vi "python_test2_quadarrays 1.vi"(0 "Time Array":dbl[](array[numeric]), 1 "Python Path on host machine":path=path "C:/Program Files (x86)/Python39-32/python.exe", 2 "Python Module Path on host machine":path=path "C:/Users/idewe/Projects/LabviewProjects/Sonomatic SQLite3 Testing/add_2_nums.py", 5 "Press Array":dbl[](array[numeric]), 7 "Temp Array":dbl[](array[numeric]), 9 "Dens Array":dbl[](array[numeric]), 11 "error in (no error)":errorcluster, 12 "Python_Function_Name":string="sum_function", 13 "Python Version":string="3.9.2") -> (4 "Python Numeric Output":dbl[](array[numeric]), 15 "error out":errorcluster)   [LabVIEW 2023]
panel:
  # "PYTHON METHOD CALL EXAMPLE"
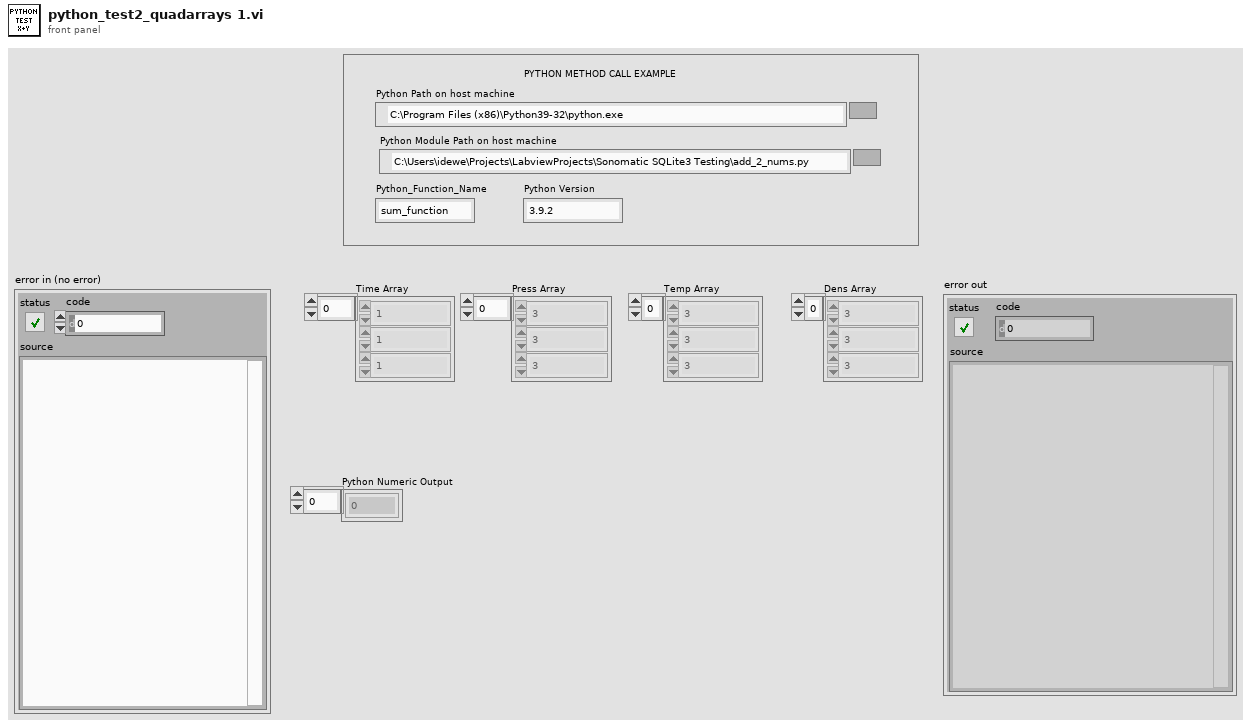
[diagram p1: front panel]
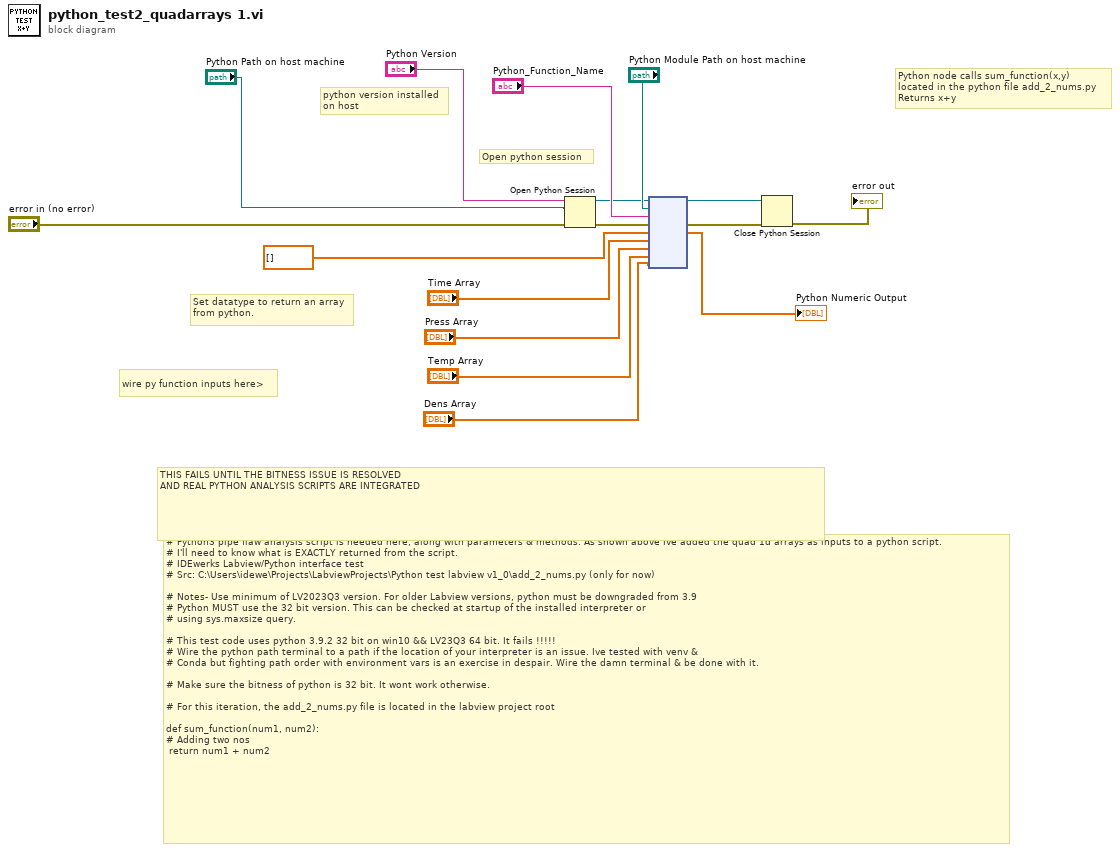
[diagram p0: block diagram]
diagram:
  # "Set datatype to return an array\nfrom python."
  # "THIS FAILS UNTIL THE BITNESS ISSUE IS RESOLVED\nAND REAL PYTHON ANALYSIS SCRIPTS ARE INTEGRATED"
  # "Open python session"
  # "Python node calls sum_function(x,y)\nlocated in the python file add_2_nums.py\nReturns x+y"
  # "wire py function inputs here>"
  # "python version installed\non host"
  # "# Python3 pipe flaw analysis script is needed here, along with parameters & methods. As shown above Ive added the quad 1d arrays as inputs to a python script.\n# I'll need to know what is EXACTLY returned from the script. \n# IDEwerks Labview/Python interface test\n# Src: C:\\Users\\idewe\\Projects\\LabviewProjects\\Python test labview v1_0\\add_2_nums.py (only for now)\n\n# Notes- Use minimum of LV2023Q3 version. For older Labview versions, python must be downgraded from 3.9\n# Python MUST use the 32 bit version. This can be checked at startup of the installed interpreter or\n# using sys.maxsize query.\n\n# This test code uses python 3.9.2 32 bit on win10 && LV23Q3 64 bit. It fails !!!!!\n# Wire the python path terminal to a path if the location of your interpreter is an issue. Ive tested with venv &\n# Conda but fighting path order with environment vars is an exercise in despair. Wire the damn terminal & be done with it.\n\n# Make sure the bitness of python is 32 bit. It wont work otherwise.\n\n# For this iteration, the add_2_nums.py file is located in the labview project root \n\ndef sum_function(num1, num2):\n# Adding two nos\n\treturn num1 + num2"
  n1 = Open Python Session(python version="Python Version", python path="Python Path on host machine", 3:"error in (no error)") -> (session out=w11:refnum<k35>, error out=w10:errorcluster)
  n2 = node(w11, "Python Module Path on host machine", "Python_Function_Name", w10, dbl[] [], "Time Array", "Press Array", "Temp Array", "Dens Array") -> (w5:refnum<k35>, w4:errorcluster, →"Python Numeric Output":dbl[])  [unwired: 4 in, 2 out]
  n3 = Close Python Session(session in=w5, error in=w4) -> (11:→"error out":errorcluster)
